vi "final.vi"() -> ()   [LabVIEW 2015]
uses:
  <vilib>/NXT/Block Support/NXT_InputPort.ctl
  <vilib>/NXT/Block Support/NXT_OutputPort.ctl
  <vilib>/NXT/Dual Mode Library/Sensors/Sonar_cm.vi
  <vilib>/NXT/Dual Mode Library/Sensors/Light_On.vi
  <vilib>/NXT/NXTIO Xnodes/NXTIONodeSubVIs/NXTMoveMotors.vi
  <vilib>/NXT/Dual Mode Library/Waits/Wait_Num.vi
  <vilib>/NXT/NXTIO Xnodes/AddressXNode/NXTIOAddress.xnode
  <vilib>/NXT/Subs/LVHSConnector.ctl
  <vilib>/NXT/NXTIO Xnodes/NXTIOXNode/NXTIO.xnode
  <vilib>/NXT/LegoClasses/BrickReference/BrickReference.lvclass
panel:
  in  "Port (Port 4)":T1=3 items=["Port 1", "Port 2", "Port 3", "Port 4"]
  in  "Port (Port 3) 3":T1=2 items=["Port 1", "Port 2", "Port 3", "Port 4"]
  in  "Port (Port 3) 4":T1=2 items=["Port 1", "Port 2", "Port 3", "Port 4"]
  in  "Power/Speed 13":i8=75
  in  "Power/Speed 10":i8=75
  in  "Power/Speed 8":i8=75
  in  "Power/Speed 17":i8=75
  in  "Power/Speed 16":i8=75
  in  "Power/Speed 15":i8=75
  in  "Power/Speed 11":i8=75
  in  "Power/Speed 12":i8=75
  in  "Power/Speed 14":i8=75
  in  "Port (Port 3)":T1=2 items=["Port 1", "Port 2", "Port 3", "Port 4"]
  in  "Port (Port 3) 2":T1=2 items=["Port 1", "Port 2", "Port 3", "Port 4"]
  in  "Power/Speed 6":i8=75
  in  "Power/Speed 9":i8=75
  in  "Power/Speed 4":i8=75
  in  "Power/Speed 5":i8=75
  in  "stop":bool
  in  "Power/Speed 3":i8=75
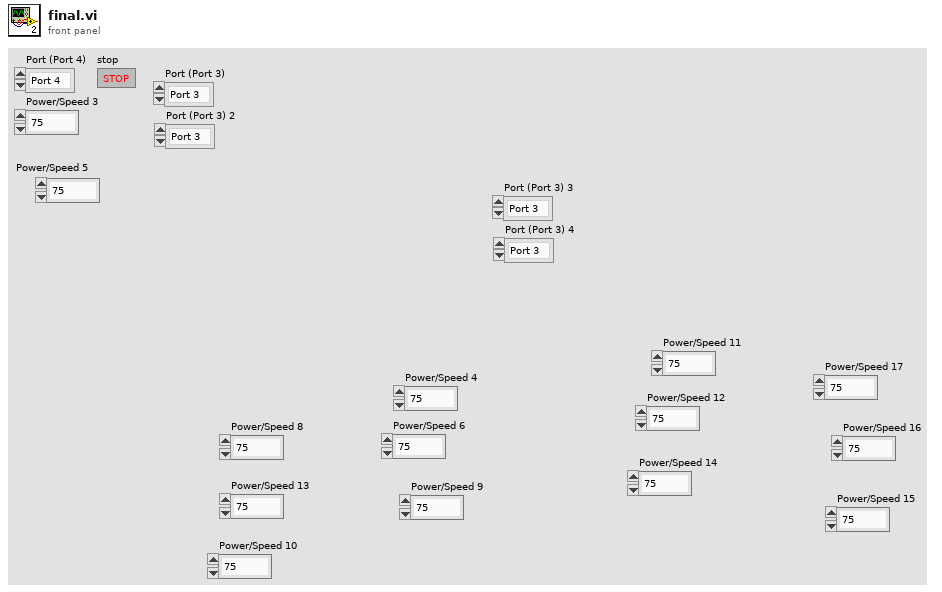
[diagram p1: front panel]
types:
  T1 = typedef "NXT_InputPort.ctl" = u32
  T2 = typedef "NXT_OutputPort.ctl" = u8
  T3 = cluster{"Output Port":T2, "Output Port 2":T2, "Output Port 3":T2}
  T4 = typedef "LVHSConnector.ctl" = refnum<class "BrickReference.lvclass">
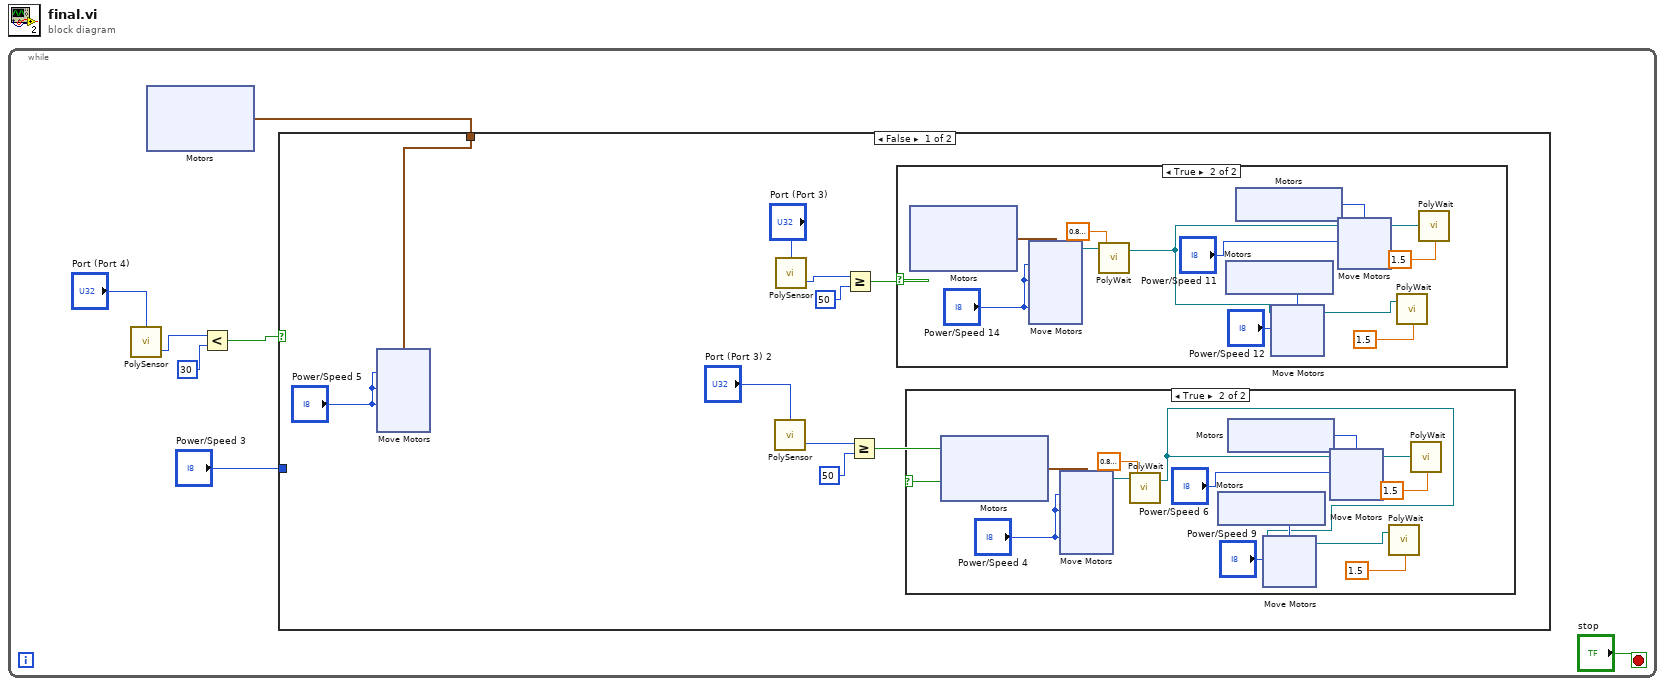
[diagram p0: block diagram]
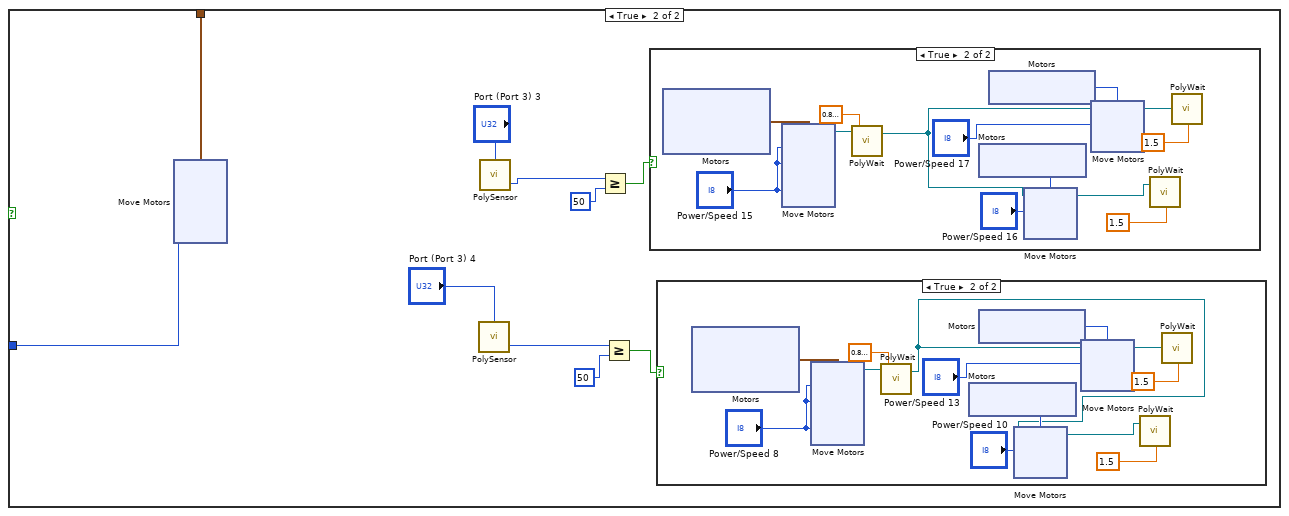
[diagram p4: hidden frame]
diagram:
  n1 = while {
    stop <- "stop" stop-if-true
    n2 = call-poly <vilib>:"PolySensor.vi"("Port (Port 4)"="Port (Port 4)") -> ("Distance (cm)"=w4:i16)  [unwired: 2 in, 1 out]
    n3 = xnode "Motors"() -> ("Motor"=w2:cluster{"Port":T2, "Port":T2, "Port":T2})
    n4 = Less?(x=w4, y=i16 30) -> (x < y?=w5:bool)
    n5 = case shown="False" w5 {
      tunnel: w2 -> [w10 w115]
      tunnel: "Power/Speed 3" -> [_ w114]
      frame False {
        n6 = xnode "Move Motors"("Power/Speed 3"="Power/Speed 5", "Power/Speed 2"="Power/Speed 5", "Power/Speed 1"="Power/Speed 5", "Motors"=w10) -> ()  [unwired: 1 in, 1 out]
        n7 = call-poly <vilib>:"PolySensor.vi"("Port (Port 3)"="Port (Port 3) 2") -> ("Scaled Value"=w13:i16)  [unwired: 2 in, 1 out]
        n8 = call-poly <vilib>:"PolySensor.vi"("Port (Port 3)"="Port (Port 3)") -> ("Scaled Value"=w17:i16)  [unwired: 2 in, 1 out]
        n9 = Greater Or Equal?(x=w17, y=i16 50) -> (x >= y?=w15:bool)
        n10 = Greater Or Equal?(x=w13, y=i16 50) -> (x >= y?=w11:bool)
        n11 = case shown="True" w15 {
          frame False {
          }
          frame True {
            n12 = xnode "Motors"() -> ("Motor"=w71:cluster{"Port":T2, "Port":T2, "Port":T2})
            n13 = xnode "Move Motors"("Power/Speed 3"="Power/Speed 14", "Power/Speed 2"="Power/Speed 14", "Power/Speed 1"="Power/Speed 14", "Motors"=w71) -> ("NXT/EV3"=w69:T4)  [unwired: 1 in]
            n14 = call-poly <vilib>:"PolyWait.vi"("Time (1 sec)"=sgl 0.8, "NXT/EV3"=w69) -> ("NXT/EV3"=w67:T4)  [unwired: 2 in]
            n15 = xnode "Motors"() -> ("Motor"=w76:T2)
            n16 = xnode "Motors"() -> ("Motor"=w79:T2)
            n17 = xnode "Move Motors"("Power/Speed 1"="Power/Speed 12", "Motors"=w76, "NXT/EV3"=w67) -> ("NXT/EV3"=w72:T4)
            n18 = xnode "Move Motors"("Power/Speed 1"="Power/Speed 11", "Motors"=w79, "NXT/EV3"=w67) -> ("NXT/EV3"=w78:T4)
            n19 = call-poly <vilib>:"PolyWait.vi"("Time (1 sec)"=sgl 1.5, "NXT/EV3"=w72) -> ()  [unwired: 2 in, 1 out]
            n20 = call-poly <vilib>:"PolyWait.vi"("Time (1 sec)"=sgl 1.5, "NXT/EV3"=w78) -> ()  [unwired: 2 in, 1 out]
          }
        }
        n21 = case shown="True" w11 {
          frame False {
          }
          frame True {
            n22 = xnode "Motors"() -> ("Motor"=w32:cluster{"Port":T2, "Port":T2, "Port":T2})
            n23 = xnode "Move Motors"("Power/Speed 3"="Power/Speed 4", "Power/Speed 2"="Power/Speed 4", "Power/Speed 1"="Power/Speed 4", "Motors"=w32) -> ("NXT/EV3"=w30:T4)  [unwired: 1 in]
            n24 = call-poly <vilib>:"PolyWait.vi"("Time (1 sec)"=sgl 0.8, "NXT/EV3"=w30) -> ("NXT/EV3"=w28:T4)  [unwired: 2 in]
            n25 = xnode "Motors"() -> ("Motor"=w37:T2)
            n26 = xnode "Motors"() -> ("Motor"=w40:T2)
            n27 = xnode "Move Motors"("Power/Speed 1"="Power/Speed 9", "Motors"=w37, "NXT/EV3"=w28) -> ("NXT/EV3"=w33:T4)
            n28 = xnode "Move Motors"("Power/Speed 1"="Power/Speed 6", "Motors"=w40, "NXT/EV3"=w28) -> ("NXT/EV3"=w39:T4)
            n29 = call-poly <vilib>:"PolyWait.vi"("Time (1 sec)"=sgl 1.5, "NXT/EV3"=w33) -> ()  [unwired: 2 in, 1 out]
            n30 = call-poly <vilib>:"PolyWait.vi"("Time (1 sec)"=sgl 1.5, "NXT/EV3"=w39) -> ()  [unwired: 2 in, 1 out]
          }
        }
      }
      frame True {
        n31 = xnode "Move Motors"("Power/Speed 3"=w114, "Power/Speed 2"=w114, "Power/Speed 1"=w114, "Motors"=w115) -> ()  [unwired: 1 in, 1 out]
        n32 = call-poly <vilib>:"PolySensor.vi"("Port (Port 3)"="Port (Port 3) 4") -> ("Scaled Value"=w109:i16)  [unwired: 2 in, 1 out]
        n33 = call-poly <vilib>:"PolySensor.vi"("Port (Port 3)"="Port (Port 3) 3") -> ("Scaled Value"=w112:i16)  [unwired: 2 in, 1 out]
        n34 = Greater Or Equal?(x=w112, y=i16 50) -> (x >= y?=w106:bool)
        n35 = Greater Or Equal?(x=w109, y=i16 50) -> (x >= y?=w107:bool)
        n36 = case shown="True" w106 {
          frame False {
          }
          frame True {
            n37 = xnode "Motors"() -> ("Motor"=w120:cluster{"Port":T2, "Port":T2, "Port":T2})
            n38 = xnode "Move Motors"("Power/Speed 3"="Power/Speed 15", "Power/Speed 2"="Power/Speed 15", "Power/Speed 1"="Power/Speed 15", "Motors"=w120) -> ("NXT/EV3"=w118:T4)  [unwired: 1 in]
            n39 = call-poly <vilib>:"PolyWait.vi"("Time (1 sec)"=sgl 0.8, "NXT/EV3"=w118) -> ("NXT/EV3"=w116:T4)  [unwired: 2 in]
            n40 = xnode "Motors"() -> ("Motor"=w125:T2)
            n41 = xnode "Motors"() -> ("Motor"=w128:T2)
            n42 = xnode "Move Motors"("Power/Speed 1"="Power/Speed 16", "Motors"=w125, "NXT/EV3"=w116) -> ("NXT/EV3"=w121:T4)
            n43 = xnode "Move Motors"("Power/Speed 1"="Power/Speed 17", "Motors"=w128, "NXT/EV3"=w116) -> ("NXT/EV3"=w127:T4)
            n44 = call-poly <vilib>:"PolyWait.vi"("Time (1 sec)"=sgl 1.5, "NXT/EV3"=w121) -> ()  [unwired: 2 in, 1 out]
            n45 = call-poly <vilib>:"PolyWait.vi"("Time (1 sec)"=sgl 1.5, "NXT/EV3"=w127) -> ()  [unwired: 2 in, 1 out]
          }
        }
        n46 = case shown="True" w107 {
          frame False {
          }
          frame True {
            n47 = xnode "Motors"() -> ("Motor"=w159:cluster{"Port":T2, "Port":T2, "Port":T2})
            n48 = xnode "Move Motors"("Power/Speed 3"="Power/Speed 8", "Power/Speed 2"="Power/Speed 8", "Power/Speed 1"="Power/Speed 8", "Motors"=w159) -> ("NXT/EV3"=w157:T4)  [unwired: 1 in]
            n49 = call-poly <vilib>:"PolyWait.vi"("Time (1 sec)"=sgl 0.8, "NXT/EV3"=w157) -> ("NXT/EV3"=w155:T4)  [unwired: 2 in]
            n50 = xnode "Motors"() -> ("Motor"=w164:T2)
            n51 = xnode "Motors"() -> ("Motor"=w167:T2)
            n52 = xnode "Move Motors"("Power/Speed 1"="Power/Speed 10", "Motors"=w164, "NXT/EV3"=w155) -> ("NXT/EV3"=w160:T4)
            n53 = xnode "Move Motors"("Power/Speed 1"="Power/Speed 13", "Motors"=w167, "NXT/EV3"=w155) -> ("NXT/EV3"=w166:T4)
            n54 = call-poly <vilib>:"PolyWait.vi"("Time (1 sec)"=sgl 1.5, "NXT/EV3"=w160) -> ()  [unwired: 2 in, 1 out]
            n55 = call-poly <vilib>:"PolyWait.vi"("Time (1 sec)"=sgl 1.5, "NXT/EV3"=w166) -> ()  [unwired: 2 in, 1 out]
          }
        }
      }
    }
  }
